vi "Get Array Data Size.vi"(8 "error in (no error)":errorcluster, 10 "Data String":u8[](array[numeric]), 11 "Type Descriptor":i16[](array[numeric])) -> (0 "error out":errorcluster, 2 "Array Data Size":i32)   [LabVIEW 2017, in "Composition.lvlib"]
doc: "Gets the data size of an array of any type."
uses:
  Composition.lvlib
  Get Data Type.vi/2a0888ac-0230-421b-a610-ddb651202d87.vi
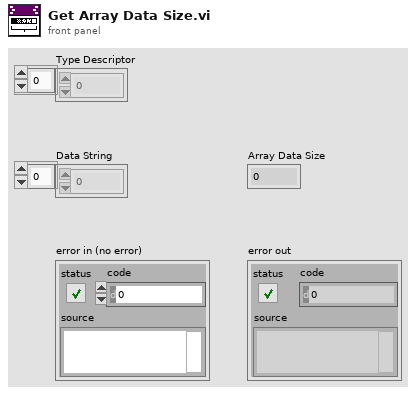
[diagram p1: front panel]
types:
  T1 = typedef "Composition.lvlib/Data Type.ctl" = enum16{"Void", "I8", "I16", "I32", "I64", "U8", "U16", "U32", "U64", "SGL", "DBL", "EXT", "CSG", "CDB", "CXT", "0x0F", "0x10", "0x11", "0x12", "0x13", "0x14", "Enum U8", "Enum U16", "Enum U32", "0x18", "SGL Physical", "DBL Physical", "EXT Physical", "CSG Physical", "CDB Physical", "CXT Physical", "0x1F", "Boolean U16", "Boolean U8", "0x22", "0x23", "0x24", "0x25", "0x26", "0x27", "0x28", "0x29", "0x2A", "0x2B", "0x2C", "0x2D", "0x2E", "0x2F", "String", "0x31", "Path", "Picture", "CString", "PString", "0x36", "Tag", "0x38", "0x39", "0x3A", "0x3B", "0x3C", "0x3D", "0x3E", "SubString", "Array", "Array Data Ptr", "0x42", "0x43", "0x44", "0x45", "0x46", "0x47", "0x48", "0x49", "0x4A", "0x4B", "0x4C", "0x4D", "0x4E", "SubArray", "Cluster", "0x51", "0x52", "Variant", "Waveform", "0x55", "0x56", "0x57", "0x58", "0x59", "0x5A", "0x5B", "0x5C", "0x5D", "CFX", "FXP", "Block", "Type Block", "Void Block", "Aligned Block", "Repeated Block", "Alignment Marker", "0x66", "0x67", "0x68", "0x69", "0x6A", "0x6B", "0x6C", "0x6D", "0x6E", "0x6F", "Refnum", "0x71", "0x72", "Set Collection", "Map Collection", "0x75", "0x76", "0x77", "0x78", "0x79", "0x7A", "0x7B", "0x7C", "0x7D", "0x7E", "0x7F", "Ptr", "0x81", "0x82", "Ptr to", "EXT Data", "0x85", "0x86", "0x87", "0x88", "0x89", "0x8A", "0x8B", "0x8C", "0x8D", "0x8E", "0x8F", "0x90", "0x91", "0x92", "0x93", "0x94", "0x95", "0x96", "0x97", "0x98", "0x99", "0x9A", "0x9B", "0x9C", "0x9D", "0x9E", "0x9F", "Array Interface", "Interface to Data", "0xA2", "0xA3", "0xA4", "0xA5", "0xA6", "0xA7", "0xA8", "0xA9", "0xAA", "0xAB", "0xAC", "0xAD", "0xAE", "0xAF", "0xB0", "0xB1", "0xB2", "0xB3", "0xB4", "0xB5", "0xB6", "0xB7", "0xB8", "0xB9", "0xBA", "0xBB", "0xBC", "0xBD", "0xBE", "0xBF", "0xC0", "0xC1", "0xC2", "0xC3", "0xC4", "0xC5", "0xC6", "0xC7", "0xC8", "0xC9", "0xCA", "0xCB", "0xCC", "0xCD", "0xCE", "0xCF", "0xD0", "0xD1", "0xD2", "0xD3", "0xD4", "0xD5", "0xD6", "0xD7", "0xD8", "0xD9", "0xDA", "0xDB", "0xDC", "0xDD", "0xDE", "0xDF", "0xE0", "0xE1", "0xE2", "0xE3", "0xE4", "0xE5", "0xE6", "0xE7", "0xE8", "0xE9", "0xEA", "0xEB", "0xEC", "0xED", "0xEE", "0xEF", "Function", "TypeDef", "PolyVI", "0xF3", "0xF4", "0xF5", "0xF6", "0xF7", "0xF8", "0xF9", "0xFA", "0xFB", "0xFC", "0xFD", "0xFE", "0xFF"}
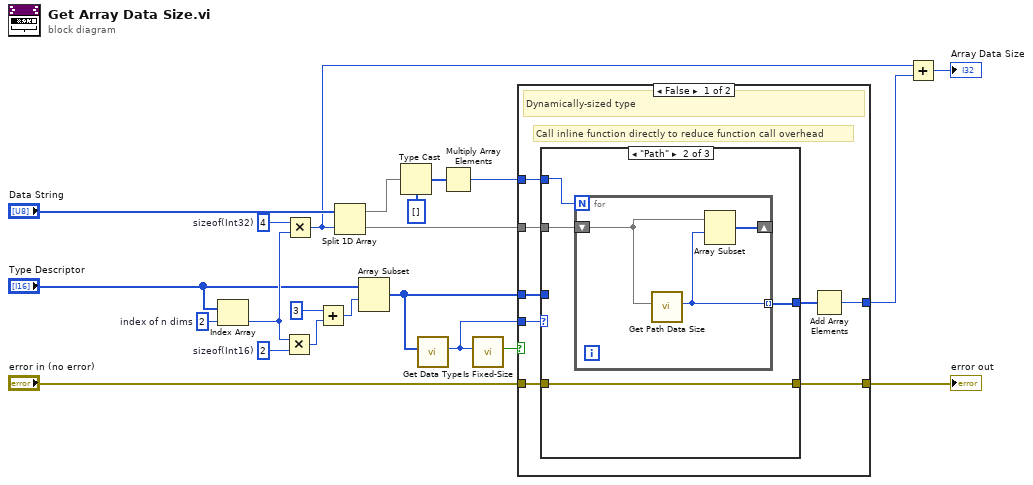
[diagram p0: block diagram]
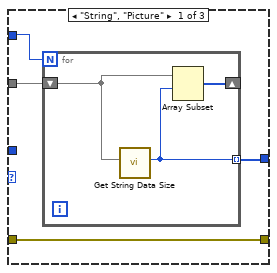
[diagram p2: hidden frame]
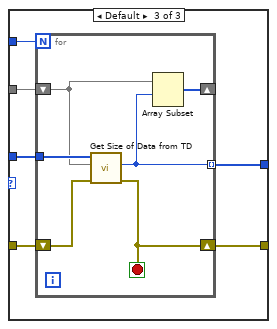
[diagram p3: hidden frame]
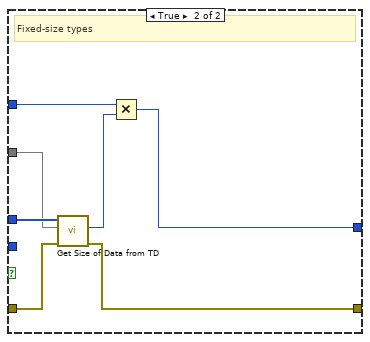
[diagram p4: hidden frame]
diagram:
  w18 = 2  # sizeof(Int16)
  w20 = 2  # index of n dims
  w19 = 4  # sizeof(Int32)
  n1 = Index Array(array="Type Descriptor", index=w20) -> (element=w16:i16)
  n2 = Multiply(x=w16, y=w18) -> (x*y=w17:i32)
  n3 = Multiply(x=w19, y=w16) -> (x*y=w7:i32)
  n4 = Add(x=3 ("index"), y=w17) -> (x+y=w15:i32)
  n5 = Split 1D Array(array="Data String", index=w7) -> (first subarray=w5:u8[], second subarray=w6:u8[])
  n6 = Array Subset(array="Type Descriptor", index=w15) -> (w11:i16[])  [unwired: 1 in]
  n7 = Type Cast(type=i32[] [], x=w5) -> (*(type *) &x=w21:i32[])
  n8 = call "Get Data Type.vi"("Type Descriptor"=w11) -> ("Data Type"=w1:T1)  [unwired: 10 in]
  n9 = Multiply Array Elements(1:w21) -> (0:w13:i32)
  n10 = call "Is Fixed-Size.vi"("Data Type"=w1) -> ("Is Fixed-Size"=w10:bool)  [unwired: 10 in]
  n11 = case shown="False" w10 {
    tunnel: w6 -> [w30 w62]
    tunnel: w13 -> [w29 w60]
    tunnel: [w27 w59] -> w12
    tunnel: w11 -> [w26 w63]
    tunnel: "error in (no error)" -> [w25 w58]
    tunnel: [w24 w57] -> w2
    tunnel: w1 -> [w23 _]
    frame False {
      # "Call inline function directly to reduce function call overhead"
      # "Dynamically-sized type"
      n12 = case shown="\"Path\"" w23 {
        tunnel: w30 -> [w33 w40 w50]
        tunnel: w29 -> [w31 w38 w49]
        tunnel: [w32 w39 w48] -> w28
        tunnel: w26 -> [_ _ w47]
        tunnel: w25 -> [w34 w41 w46]
        tunnel: [w34 w41 w45] -> w24
        frame "String", "Picture" {
          n13 = for {
            N: w31 -> [_]
            shift-right: [w37] -> _
            shift-left: w33 -> [w36]
            tunnel: [w35] -> w32 mode=indexing
            n14 = call "Get String Data Size.vi"("Data String"=w36) -> ("Data Size"=w35:i32)  [unwired: 10 in]
            n15 = Array Subset(array=w36, index=w35) -> (w37:u8[])  [unwired: 1 in]
          }
        }
        frame "Path" {
          n16 = for {
            N: w38 -> [_]
            shift-right: [w44] -> _
            shift-left: w40 -> [w43]
            tunnel: [w42] -> w39 mode=indexing
            n17 = call "Get Path Data Size.vi"("Data String"=w43) -> ("Data Size"=w42:i32)  [unwired: 10 in]
            n18 = Array Subset(array=w43, index=w42) -> (w44:u8[])  [unwired: 1 in]
          }
        }
        frame Default {
          n19 = for {
            N: w49 -> [_]
            tunnel: w47 -> [w56]
            shift-right: [w54] -> _
            shift-left: w50 -> [w55]
            tunnel: [w53] -> w48 mode=indexing
            shift-right: [w51] -> w45
            shift-left: w46 -> [w52]
            stop <- w51 stop-if-true
            n20 = call "Get Size of Data from TD.vi"("error in (no error)"=w52, "Data String"=w55, "Type Descriptor"=w56) -> ("error out"=w51:errorcluster, "Size of Data"=w53:i32)  [unwired: 7 in]
            n21 = Array Subset(array=w55, index=w53) -> (w54:u8[])  [unwired: 1 in]
          }
        }
      }
      n22 = Add Array Elements(numeric array=w28) -> (sum=w27:i32)
    }
    frame True {
      # "Fixed-size types"
      n23 = call "Get Size of Data from TD.vi"("error in (no error)"=w58, "Data String"=w62, "Type Descriptor"=w63) -> ("error out"=w57:errorcluster, "Size of Data"=w61:i32)  [unwired: 7 in]
      n24 = Multiply(x=w60, y=w61) -> (x*y=w59:i32)
    }
  }
  "error out" <- w2
  n25 = Add(x=w7, y=w12) -> (x+y=→"Array Data Size":i32)
